vi "MTMount_getNextSample_OSS2.vi"(8 "error in (no error)":errorcluster, 11 "OSS2_Ctl":T1) -> (0 "error out":errorcluster, 2 "function return":i32, 3 "OSS2_Ctl out":T1)   [LabVIEW 2018, in "SALLV_MTMount.lvlib"]
doc: "int MTMount_shm_getNextSample_OSS2LV(MTMount_OSS2LV *OSS2_Ctl );"
uses:
  SALLV_MTMount.lvlib
  DataTypes/OSS2.ctl
  SALLV_MTMount.so
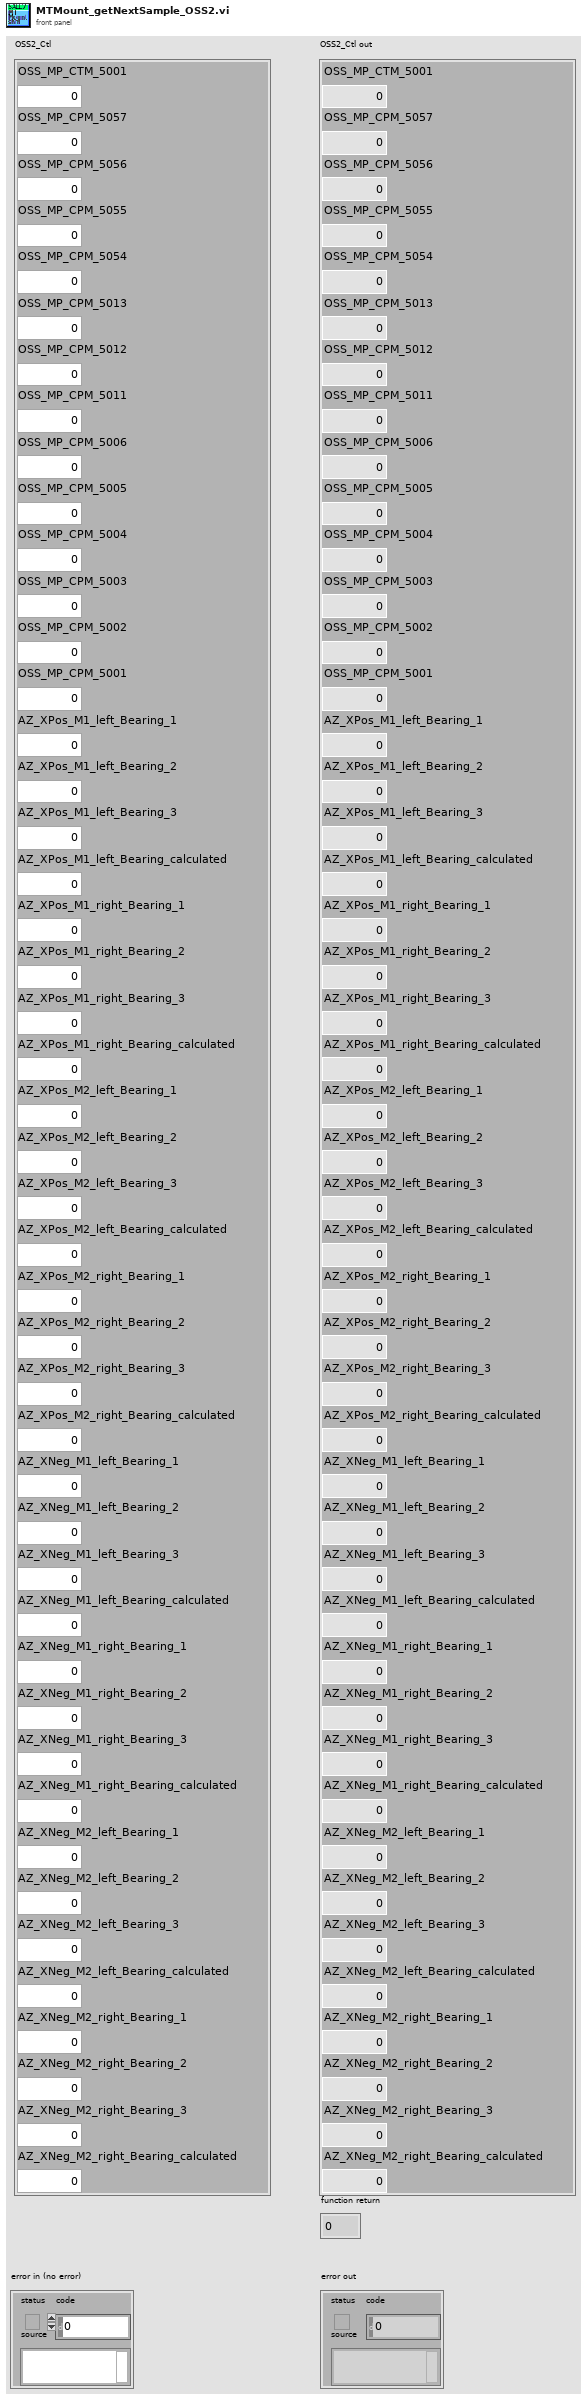
[diagram p1: front panel]
types:
  T1 = typedef "SALLV_MTMount.lvlib/OSS2.ctl" = cluster{"OSS_MP_CTM_5001":dbl, "OSS_MP_CPM_5057":dbl, "OSS_MP_CPM_5056":dbl, "OSS_MP_CPM_5055":dbl, "OSS_MP_CPM_5054":dbl, "OSS_MP_CPM_5013":dbl, "OSS_MP_CPM_5012":dbl, "OSS_MP_CPM_5011":dbl, "OSS_MP_CPM_5006":dbl, "OSS_MP_CPM_5005":dbl, "OSS_MP_CPM_5004":dbl, "OSS_MP_CPM_5003":dbl, "OSS_MP_CPM_5002":dbl, "OSS_MP_CPM_5001":dbl, "AZ_XPos_M1_left_Bearing_1":dbl, "AZ_XPos_M1_left_Bearing_2":dbl, "AZ_XPos_M1_left_Bearing_3":dbl, "AZ_XPos_M1_left_Bearing_calculated":dbl, "AZ_XPos_M1_right_Bearing_1":dbl, "AZ_XPos_M1_right_Bearing_2":dbl, "AZ_XPos_M1_right_Bearing_3":dbl, "AZ_XPos_M1_right_Bearing_calculated":dbl, "AZ_XPos_M2_left_Bearing_1":dbl, "AZ_XPos_M2_left_Bearing_2":dbl, "AZ_XPos_M2_left_Bearing_3":dbl, "AZ_XPos_M2_left_Bearing_calculated":dbl, "AZ_XPos_M2_right_Bearing_1":dbl, "AZ_XPos_M2_right_Bearing_2":dbl, "AZ_XPos_M2_right_Bearing_3":dbl, "AZ_XPos_M2_right_Bearing_calculated":dbl, "AZ_XNeg_M1_left_Bearing_1":dbl, "AZ_XNeg_M1_left_Bearing_2":dbl, "AZ_XNeg_M1_left_Bearing_3":dbl, "AZ_XNeg_M1_left_Bearing_calculated":dbl, "AZ_XNeg_M1_right_Bearing_1":dbl, "AZ_XNeg_M1_right_Bearing_2":dbl, "AZ_XNeg_M1_right_Bearing_3":dbl, "AZ_XNeg_M1_right_Bearing_calculated":dbl, "AZ_XNeg_M2_left_Bearing_1":dbl, "AZ_XNeg_M2_left_Bearing_2":dbl, "AZ_XNeg_M2_left_Bearing_3":dbl, "AZ_XNeg_M2_left_Bearing_calculated":dbl, "AZ_XNeg_M2_right_Bearing_1":dbl, "AZ_XNeg_M2_right_Bearing_2":dbl, "AZ_XNeg_M2_right_Bearing_3":dbl, "AZ_XNeg_M2_right_Bearing_calculated":dbl}
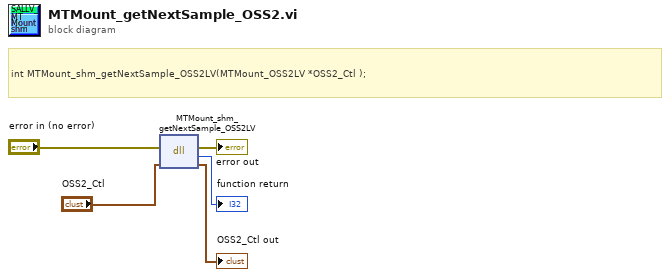
[diagram p0: block diagram]
diagram:
  # "int MTMount_shm_getNextSample_OSS2LV(MTMount_OSS2LV *OSS2_Ctl );"
  n1 = dll-call lib="home/ttsai/Document/salApiMTMount/SALLV_MTMount/SALLV_MTMount.*" fn="MTMount_shm_getNextSample_OSS2LV"(error in="error in (no error)", "OSS2_Ctl"="OSS2_Ctl") -> (error out=→"error out":errorcluster, →"function return":i32, "OSS2_Ctl"=→"OSS2_Ctl out":T1)  [unwired: 2 in, 1 out]
